vi "ToJson.vi"(8 "error in (no error)":errorcluster, 11 "Request":refnum<class "Request.lvclass">) -> (0 "error out":errorcluster, 2 "Request":string)   [LabVIEW 2015, in "Request.lvclass"]
uses:
  Request.lvclass
  JsonCluster.ctl
  Request.lvclass/Request.ctl
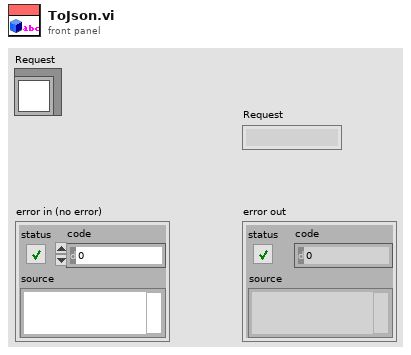
[diagram p1: front panel]
types:
  T1 = typedef "Request.lvclass/JsonCluster.ctl" = cluster{"RequestID":string, "PersonnelType":i32, "StartTime":string, "StartName":string, "AckTime":string, "AckName":string, "FulfilledTime":string, "FulfilledName":string, "Description":string, "RoomNumber":i32, "RequestType":i32, "Alarm":bool}
  T2 = typedef "Request.lvclass/PersonnelType.ctl" = u16
  T3 = typedef "Request.lvclass/RequestType.ctl" = enum16{"Specific Call To Room", "General Call To Room"}
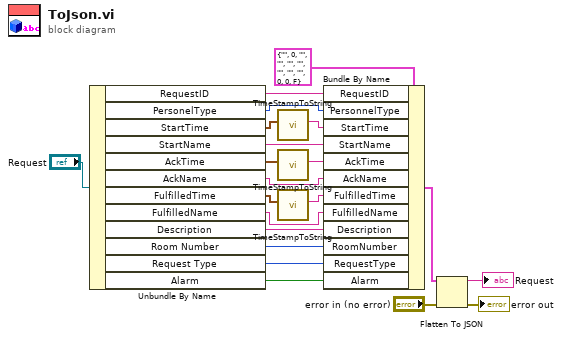
[diagram p0: block diagram]
diagram:
  n1 = Unbundle By Name("Request") -> ("RequestID"=w15:string, "PersonelType"=w14:T2, "StartTime"=w9:timestamp, "StartName"=w13:string, "AckTime"=w7:timestamp, "AckName"=w12:string, "FulfilledTime"=w5:timestamp, "FulfilledName"=w11:string, "Description"=w10:string, "Room Number"=w3:i32, "Request Type"=w2:T3, "Alarm"=w1:bool)
  n2 = call "TimeStampToString.vi"("Time Stamp"=w9) -> ("String"=w8:string)  [unwired: 9 in, 1 out]
  n3 = call "TimeStampToString.vi"("Time Stamp"=w7) -> ("String"=w6:string)  [unwired: 9 in, 1 out]
  n4 = call "TimeStampToString.vi"("Time Stamp"=w5) -> ("String"=w4:string)  [unwired: 9 in, 1 out]
  n5 = Bundle By Name(cluster=T1 {"RequestID"="", "PersonnelType"=0, "StartTime"="", "StartName"="", "AckTime"="", "AckName"="", "FulfilledTime"="", "FulfilledName"="", "Description"="", "RoomNumber"=0, "RequestType"=0, "Alarm"=FALSE} ("RequestTable"), "RequestID"=w15, "PersonnelType"=w14, "StartTime"=w8, "StartName"=w13, "AckTime"=w6, "AckName"=w12, "FulfilledTime"=w4, "FulfilledName"=w11, "Description"=w10, "RoomNumber"=w3, "RequestType"=w2, "Alarm"=w1) -> (w20:T1)
  n6 = Flatten To JSON(anything=w20, error in (no error)="error in (no error)") -> (JSON string=→"Request":string, 11:→"error out":errorcluster)  [unwired: 1 in]
